vi "Send Response.vi"(0 "reference in":refnum<class "ZMQ_slave.lvclass">, 1 "response":string, 2 "data":variant, 5 "error in (no error)":errorcluster) -> (14 "reference out":refnum<class "ZMQ_slave.lvclass">, 19 "error out":errorcluster)   [LabVIEW 2019, in "CommandResponse communication.lvlib" / "ZMQ_slave.lvclass"]
doc: "Sends response message to master. Should be called after recieving and processing command"
uses:
  ZMQ_slave.lvclass
  SubVIs/mmWave data_class/mmWave data.lvclass
  <vilib>/addons/zeromq/zmq_socket.lvclass
  CommandResponse communication.lvlib
  <vilib>/Utility/Data Type/NI_Data Type.lvlib
panel:
  out "qualified LabVIEW class name":string[](array[string])
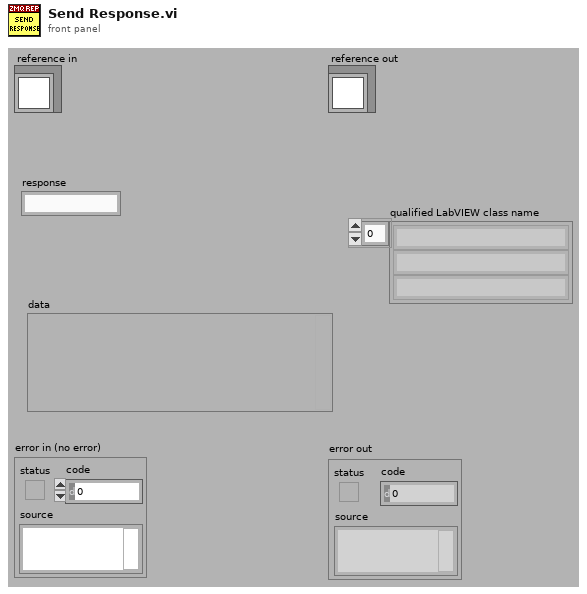
[diagram p1: front panel]
types:
  T1 = typedef "CommandResponse communication.lvlib/ZMQ_slave.lvclass/ObjectAttributes.ctl" = cluster{"ZMQ context":refnum<class "zmq_context.lvclass">, "ZMQ socket":refnum<class "zmq_socket.lvclass">, "endpoint":string}
  T2 = typedef "NI_Data Type.lvlib/Data Type.ctl" = enum8{"Invalid Type", "Void", "I8", "I16", "I32", "I64", "U8", "U16", "U32", "U64", "Single Float", "Double Float", "Extended Float", "Single Complex", "Double Complex", "Extended Complex", "Enum U8", "Enum U16", "Enum U32", "Enum U64", "Single Float With Unit", "Double Float With Unit", "Extended Float With Unit", "Single Complex with Unit", "Double Complex with Unit", "Extended Complex with Unit", "Boolean", "String", "Path", "Picture", "Tag", "Array", "Cluster", "Variant", "LV Variant", "Waveform", "Timestamp", "Digital Waveform", "Digital Data", "ExpressData", "Refnum", "External Data", "VI", "Poly VI", "LabVIEW Class Instance", "Fixed Point", "Set Collection", "Map Collection"}
  T3 = enum16{"big-endian, network order", "native, host order", "little-endian"}
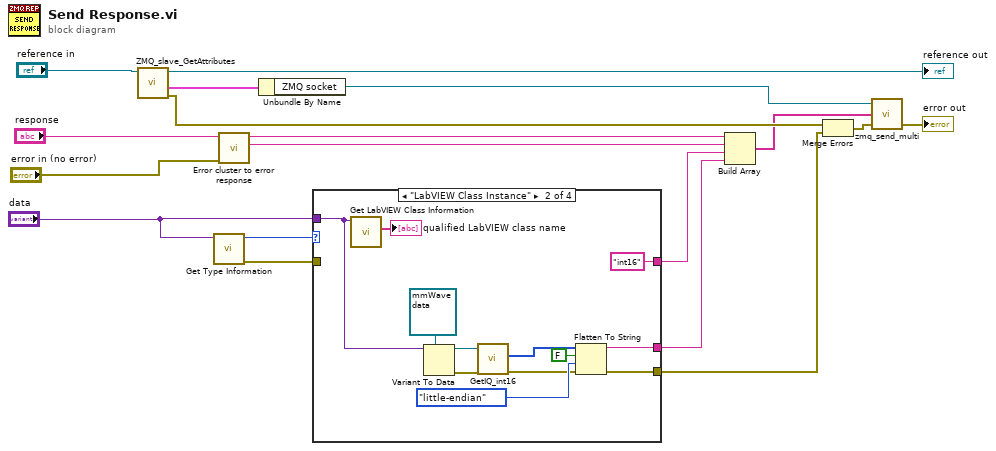
[diagram p0: block diagram]
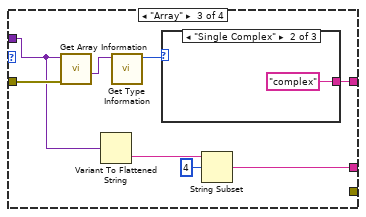
[diagram p3: hidden frame]
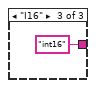
[diagram p5: hidden frame]
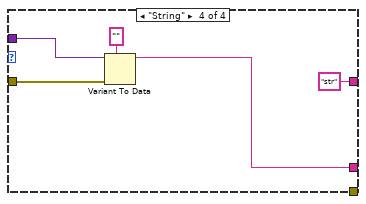
[diagram p6: hidden frame]
diagram:
  n1 = call "ZMQ_slave_GetAttributes.vi"("reference in"="reference in") -> ("error out"=w12:errorcluster, "attributes"=w16:T1, "reference out"=→"reference out":refnum<class "ZMQ_slave.lvclass">)  [unwired: 7 in, 1 out]
  n2 = call <vilib>:"Get Type Information.vi"("variant"="data") -> ("error out"=w7:errorcluster, "type"=w6:T2)  [unwired: 6 in, 3 out]
  n3 = call "Error cluster to error response.vi"("error in (no error)"="error in (no error)", "response"="response") -> ("JSON String"=w9:string, "message"=w10:string)  [unwired: 7 in, 1 out]
  n4 = Unbundle By Name(w16) -> ("ZMQ socket"=w15:refnum<class "zmq_socket.lvclass">)
  n5 = case shown="\"LabVIEW Class Instance\"" w6 {
    tunnel: w7 -> [_ _ w38 w43]
    tunnel: "data" -> [_ w28 w31 w44]
    tunnel: [_ w23 w34 w42] -> w4
    tunnel: [_ "int16" w32 "str"] -> w3
    tunnel: [_ w20 _ _] -> w1
    frame "Invalid Type", Default {
    }
    frame "LabVIEW Class Instance" {
      n6 = call <vilib>:"Get LabVIEW Class Information.vi"("variant"=w28) -> ("qualified LabVIEW class name"=→"qualified LabVIEW class name":string[])  [unwired: 8 in, 2 out]
      n7 = Variant To Data(type=refnum<class "mmWave data.lvclass"> refnum ("mmWave data"), Variant=w28) -> (data=w25:refnum<class "mmWave data.lvclass">, error out=w26:errorcluster)  [unwired: 1 in]
      n8 = call-dynamic "GetIQ_int16.vi"("error in (no error)"=w26, "reference in"=w25) -> ("error out"=w21:errorcluster, "data"=w19:i16[])  [unwired: 6 in, 2 out]
      n9 = Flatten To String(anything=w19, prepend array or string size? (T)=FALSE, byte order (0:big-endian, network order)=T3."little-endian", error in (no error)=w21) -> (data string=w23:string, error out=w20:errorcluster)  [unwired: 1 out]
    }
    frame "Array" {
      n10 = call <vilib>:"Get Array Information.vi"("error in (no error)"=w38, "variant"=w31) -> ("array element data type"=w37:variant)  [unwired: 6 in, 3 out]
      n11 = Variant To Flattened String(Variant=w31) -> (data string=w35:string)  [unwired: 1 out]
      n12 = call <vilib>:"Get Type Information.vi"("variant"=w37) -> ("type"=w33:T2)  [unwired: 6 in, 4 out]
      n13 = case shown="\"Single Complex\"" w33 {
        tunnel: [_ "complex" "int16"] -> w32
        frame "Invalid Type", Default {
        }
        frame "Single Complex" {
        }
        frame "I16" {
        }
      }
      n14 = String Subset(string=w35, offset (0)=4) -> (substring=w34:string)  [unwired: 1 in]
    }
    frame "String" {
      n15 = Variant To Data(error in=w43, type="", Variant=w44) -> (data=w42:string)  [unwired: 1 out]
    }
  }
  n16 = Build Array(w10, w9, w3, w4) -> (w8:string[])
  n17 = Merge Errors(w12, w1) -> (w2:errorcluster)
  n18 = call <vilib>:"zmq_send_multi.vi"("error in"=w2, "parts"=w8, "socket in"=w15) -> ("error out"=→"error out":errorcluster)  [unwired: 1 in, 1 out]
